vi "Test Detailed Error.vi"   [LabVIEW 2020]
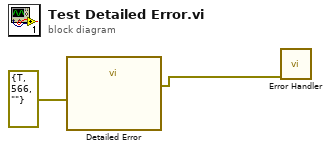
[diagram p0: block diagram]
diagram:
  n1 = call "Detailed Error"("Secondary"=errorcluster {"status"=TRUE, "code"=566, "source"=""}) -> ("detailed error"=w2:errorcluster)  [unwired: 14 in]
  n2 = call "Error Handler.vi"("error in (no error)"=w2) -> ()  [unwired: 12 in, 3 out]
